vi "Periodic Tasks.vi"(8 "error in":errorcluster) -> ()   [LabVIEW 2018]
doc: "This VI runs in parallel to other tasks. It can contain as many user-defined periodic loops as you need. These can carry out PID or other sorts of timed response."
uses:
  <vilib>/Rock Robotics/WPI/DriverStation/WPI_DriverStationRobotMode2.ctl
  <vilib>/Rock Robotics/WPI/Utilities/WPI_GetSetVariantRefNum.vi
  Robot Global Data.vi
  <vilib>/Rock Robotics/WPI/ThirdParty/Phoenix-LabVIEW/Motor Controller/Get/CTRE_Phoenix_MotorController_GetQuadratureData.vi
panel:
  out "XY Graph":cluster{"Y":dbl[], "Y":dbl[]}[](graph)
  out "Y position":dbl
  out "X position":dbl
  out "status":dbl
  out "Yaw":dbl
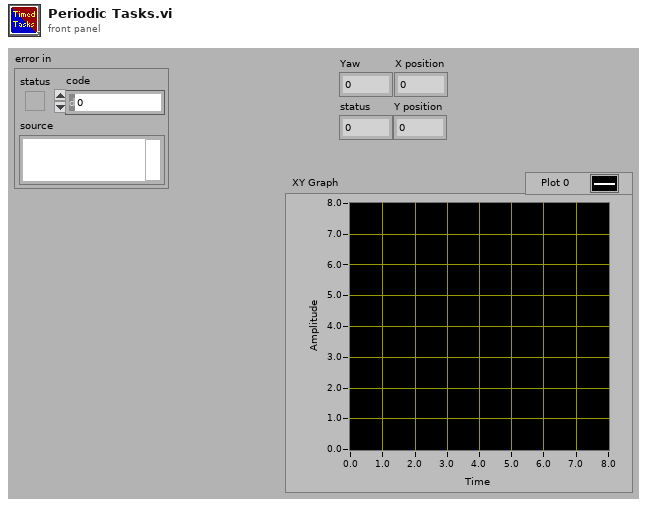
[diagram p1: front panel]
types:
  T1 = typedef "WPI_JoystickDevRef.ctl" = cluster{"Device":T2}
  T2 = typedef "WPI_JoystickDeviceEnum.ctl" = enum16{"USB 0", "USB 1", "USB 2", "USB 3", "USB 4", "USB 5"}
  T3 = typedef "WPI_RobotDriveDevRef.ctl" = cluster{"DevStatus":errorcluster, "Motors[]":T4[], "Square Inputs":bool, "Max Output":dbl}
  T4 = typedef "WPI_MotorControlDeviceRef.ctl" = cluster{"DeviceStatus":errorcluster, "Type":T5, "PWM":cluster{"PWM Channel":T6, "DeadBand":T7}, "CAN":cluster{"Device Number":u8, "SetOutput VI Ref":variant, "GetOutput VI Ref":variant, "Enable VI Ref":variant, "Disable VI Ref":variant, "Data":variant}, "Invert":bool, "DIO PWM":cluster{"PWM \"Enable\" Channel":T6, "DIOChannel":T8, "PWM Rate":dbl}}
  T5 = typedef "WPI_MotorControlType.ctl" = enum16{"PWM", "CAN", "DIO PWM"}
  T6 = typedef "FPGA_DIOPWMChannel.ctl" = enum8{"PWM 0", "PWM 1", "PWM 2", "PWM 3", "PWM 4", "PWM 5", "PWM 6", "PWM 7", "PWM 8", "PWM 9", "PWM MXP 0", "PWM MXP 1", "PWM MXP 2", "PWM MXP 3", "PWM MXP 4", "PWM MXP 5", "PWM MXP 6", "PWM MXP 7", "PWM MXP 8", "PWM MXP 9", "Invalid"}
  T7 = typedef "WPI_PWMDeadband.ctl" = cluster{"Name":string, "maxPositivePwm":i32, "minPositivePwm":i32, "centerPwm":i32, "maxNegativePwm":i32, "minNegativePwm":i32, "angularRange":u16}
  T8 = typedef "FPGA_DIOChannel.ctl" = enum8{"DIO 0", "DIO 1", "DIO 2", "DIO 3", "DIO 4", "DIO 5", "DIO 6", "DIO 7", "DIO 8", "DIO 9", "DIO MXP 0", "DIO MXP 1", "DIO MXP 2", "DIO MXP 3", "DIO MXP 4", "DIO MXP 5", "DIO MXP 6", "DIO MXP 7", "DIO MXP 8", "DIO MXP 9", "DIO MXP 10", "DIO MXP 11", "DIO MXP 12", "DIO MXP 13", "DIO MXP 14", "DIO MXP 15", "SPI Port CS1", "SPI Port CS2", "SPI Port CS3", "SPI Port MISO", "SPI Port MOSI", "Invalid"}
  T9 = cluster{"JoystickDevRef":T1, "RobotDriveDevRef":T3}
  T10 = typedef "WPI_DriverStationRobotMode2.ctl" = enum16{"Autonomous Disabled", "Autonomous Enabled", "Teleop Disabled", "Teleop Enabled", "Disconnected", "Finish", "Test Disabled", "Test Enabled", "Emergency Stopped"}
  T11 = cluster{"Yaw":dbl, "Roll":dbl, "Pitch":dbl, "Heading":dbl, "Fused Heading":dbl}
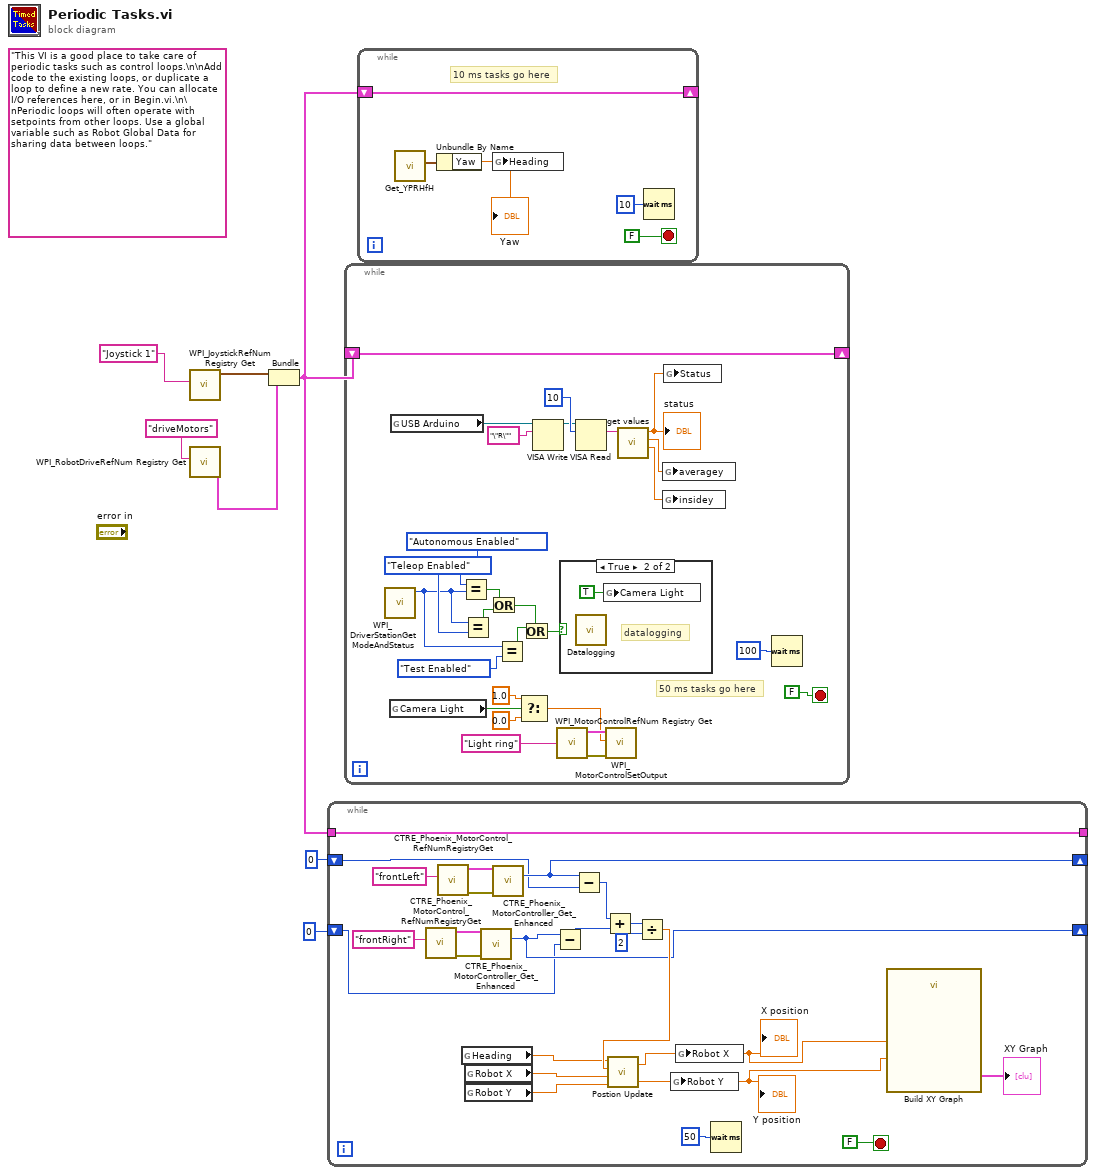
[diagram p0: block diagram]
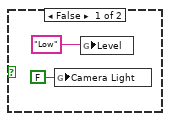
[diagram p2: hidden frame]
diagram:
  (unwired) "This VI is a good place to take care of periodic tasks such as control loops.\n\nAdd code to the existing loops, or duplicate a loop to define a new rate. You can allocate I/O references here, or in Begin.vi.\n\nPeriodic loops will often operate with setpoints from other loops. Use a global variable such as Robot Global Data for sharing data between loops."
  n1 = call <vilib>:"WPI_JoystickRefNum Registry Get.vi"("refnum name"="Joystick 1") -> ("JoystickDevRef"=w5:T1)  [unwired: 1 in, 9 out]
  n2 = call <vilib>:"WPI_RobotDriveRefNum Registry Get.vi"("refnum name"="driveMotors") -> ("RobotDriveDevRef"=w4:T3)  [unwired: 1 in, 9 out]
  n3 = Bundle("JoystickDevRef"=w5, "RobotDriveDevRef"=w4) -> (w3:T9)  [unwired: 1 out]
  n4 = while {
    tunnel: w3 -> [w31]
    tunnel: [w31] -> _
    shift-right: [w14] -> _
    shift-left: 0 -> [w13]
    shift-right: [w12] -> _
    shift-left: 0 -> [w11]
    stop <- FALSE stop-if-true
    n5 = call <vilib>:"CTRE_Phoenix_MotorControl_RefNumRegistryGet.vi"("refnum name"="frontRight") -> ("error out"=w25:errorcluster, "PhoenixMotorControlDevRef"=w23:T4)  [unwired: 9 in]
    n6 = call <vilib>:"CTRE_Phoenix_MotorControl_RefNumRegistryGet.vi"("refnum name"="frontLeft") -> ("error out"=w27:errorcluster, "PhoenixMotorControlDevRef"=w28:T4)  [unwired: 9 in]
    n7 = global read "Robot Global Data.vi" "Heading"() -> (w19:dbl)
    n8 = global read "Robot Global Data.vi" "Robot X"() -> (w29:dbl)
    n9 = global read "Robot Global Data.vi" "Robot Y"() -> (w30:dbl)
    n10 = call-poly <vilib>:"CTRE_Phoenix_MotorController_Get_Enhanced.vi"("PhoenixMotorControlDevRef"=w23, "error in"=w25) -> ("Quadrature Position"=w12:i32)  [unwired: 10 in, 3 out]
    n11 = call-poly <vilib>:"CTRE_Phoenix_MotorController_Get_Enhanced.vi"("PhoenixMotorControlDevRef"=w28, "error in"=w27) -> ("Quadrature Position"=w14:i32)  [unwired: 10 in, 3 out]
    n12 = Subtract(x=w12, y=w11) -> (x-y=w16:i32)
    n13 = Subtract(x=w14, y=w13) -> (x-y=w15:i32)
    n14 = Add(x=w15, y=w16) -> (x+y=w22:i32)
    n15 = Divide(x=w22, y=2) -> (x/y=w20:dbl)
    n16 = call "Postion Update.vi"("Y position in"=w30, "X position in"=w29, "Distance"=w20, "Heading"=w19) -> ("Y position"=w8:dbl, "X position"=w9:dbl)
    "X position" <- w9
    "Y position" <- w8
    n17 = global write "Robot Global Data.vi" "Robot Y"(w8) -> ()
    n18 = global write "Robot Global Data.vi" "Robot X"(w9) -> ()
    n19 = Wait (ms)(milliseconds to wait=u32 50) -> ()  [unwired: 1 out]
    n20 = call "Build XY Graph"("Y Input"=w8, "X Input"=w9) -> ("XY Graph"=→"XY Graph":cluster{"X":dbl[], "Y":dbl[]}[])  [unwired: 8 in, 1 out]
  }
  n21 = while {
    shift-right: [w56] -> _
    shift-left: w3 -> [w56]
    stop <- FALSE stop-if-true
    # "50 ms tasks go here"
    n22 = call <vilib>:"WPI_DriverStationGetModeAndStatus.vi"() -> ("Robot Mode"=w46:T10)  [unwired: 10 in, 1 out]
    n23 = global read "Robot Global Data.vi" "Camera Light"() -> (w36:bool)
    n24 = global read "Robot Global Data.vi" "USB Arduino"() -> (w41:refnum<visa-resource-name>)
    n25 = Equal?(x=WPI_DriverStationRobotMode2."Autonomous Enabled" ("Robot Mode"), y=w46) -> (x = y?=w49:bool)
    n26 = Equal?(x=w46, y=WPI_DriverStationRobotMode2."Teleop Enabled" ("Robot Mode")) -> (x = y?=w43:bool)
    n27 = Or(x=w49, y=w43) -> (x .or. y?=w42:bool)
    n28 = Equal?(x=w46, y=WPI_DriverStationRobotMode2."Test Enabled" ("Robot Mode")) -> (x = y?=w47:bool)
    n29 = Select(t=1.0, s=w36, f=0.0) -> (s? t:f=w33:dbl)
    n30 = Or(x=w47, y=w42) -> (x .or. y?=w44:bool)
    n31 = VISA Write(VISA resource name=w41, write buffer="\"R\"") -> (VISA resource name out=w40:refnum<visa-resource-name>)  [unwired: 1 in, 2 out]
    n32 = call <vilib>:"WPI_MotorControlRefNum Registry Get.vi"("refnum name"="Light ring") -> ("error out"=w38:errorcluster, "MotorControlDevRef"=w37:T4)  [unwired: 9 in]
    n33 = case shown="True" w44 {
      frame False {
        n34 = global write "Robot Global Data.vi" "Camera Light"(FALSE ("Camera Light")) -> ()
        n35 = global write "Robot Global Data.vi" "Level"("Low" ("Level")) -> ()
      }
      frame True {
        # "datalogging"
        n36 = call "Datalogging.vi"() -> ()  [unwired: 12 in]
        n37 = global write "Robot Global Data.vi" "Camera Light"(TRUE ("Camera Light")) -> ()
      }
    }
    n38 = VISA Read(VISA resource name=w40, byte count=u32 10) -> (read buffer=w52:string)  [unwired: 1 in, 3 out]
    n39 = call <vilib>:"WPI_MotorControlSetOutput.vi"("error in (no error)"=w38, "Output"=w33, "MotorControlDevRef"=w37) -> ()  [unwired: 6 in, 3 out]
    n40 = call "get values.vi"("USB In"=w52) -> ("insidex (0-319)"=w53:dbl, "averagex (0-319)"=w54:dbl, "status"=w55:dbl)  [unwired: 8 in]
    "status" <- w55
    n41 = global write "Robot Global Data.vi" "averagey"(w54) -> ()
    n42 = global write "Robot Global Data.vi" "insidey"(w53) -> ()
    n43 = global write "Robot Global Data.vi" "Status"(w55) -> ()
    n44 = Wait (ms)(milliseconds to wait=u32 100) -> ()  [unwired: 1 out]
  }
  n45 = while {
    shift-right: [w64] -> _
    shift-left: w3 -> [w64]
    stop <- FALSE stop-if-true
    # "10 ms tasks go here"
    n46 = call <vilib>:"Get_YPRHfH.vi"() -> ("YRPHfH"=w63:T11)  [unwired: 11 in]
    n47 = Unbundle By Name(w63) -> ("Yaw"=w62:dbl)
    "Yaw" <- w62
    n48 = global write "Robot Global Data.vi" "Heading"(w62) -> ()
    n49 = Wait (ms)(milliseconds to wait=u32 10) -> ()  [unwired: 1 out]
  }
